vi "New.vi"(6 "Delimiters":T1={"Close"="}}", "Open"="{{"}, 8 "Error In":errorcluster, 11 "Key":string) -> (0 "Error Out":errorcluster, 3 "Begin Section":refnum<class "BeginSection.lvclass">)   [LabVIEW 2018, in "Toolkit.lvlib" / "Tokens.lvlib" / "BeginSection.lvclass"]
doc: "Creates a new Begin Section object."
uses:
  BeginSection.lvclass
  Type Definitions/Delimiters.ctl
  Toolkit.lvlib
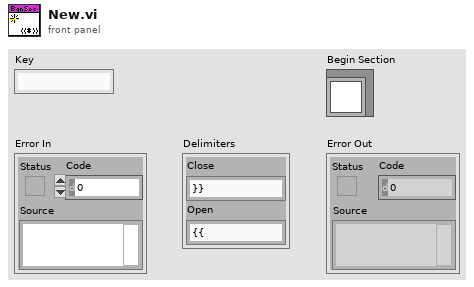
[diagram p1: front panel]
types:
  T1 = typedef "Toolkit.lvlib/Delimiters.ctl" = cluster{"Close":string, "Open":string}
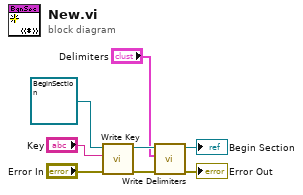
[diagram p0: block diagram]
diagram:
  n1 = call-dynamic "Write Key.vi"("Error In"="Error In", "Key"="Key", "Keyable In"=refnum<class "BeginSection.lvclass"> refnum ("Mustache.lvlib:Tokens.lvlib:BeginSection.lvclass")) -> ("Error Out"=w3:errorcluster, "Keyable Out"=w5:refnum<class "BeginSection.lvclass">)  [unwired: 7 in]
  n2 = call-dynamic "Write Delimiters.vi"("Error In"=w3, "Delimiters"="Delimiters", "Token In"=w5) -> ("Error Out"=→"Error Out":errorcluster, "Token Out"=→"Begin Section":refnum<class "BeginSection.lvclass">)  [unwired: 7 in]
